vi "SkySparkCallForgetAcq.vi"(8 "error in (no error)":errorcluster, 11 "SkySparkDevice in":refnum<class "SkySparkDevice.lvclass">) -> (0 "error out":errorcluster, 2 "FGV_Cluster Output":T1, 3 "SkySparkDevice out":refnum<class "SkySparkDevice.lvclass">)   [LabVIEW 2020, in "SkySparkDevice.lvclass"]
uses:
  SkySparkDevice.lvclass
  FGV_TypeDef.ctl
  FGVFunctionTypeDef.ctl
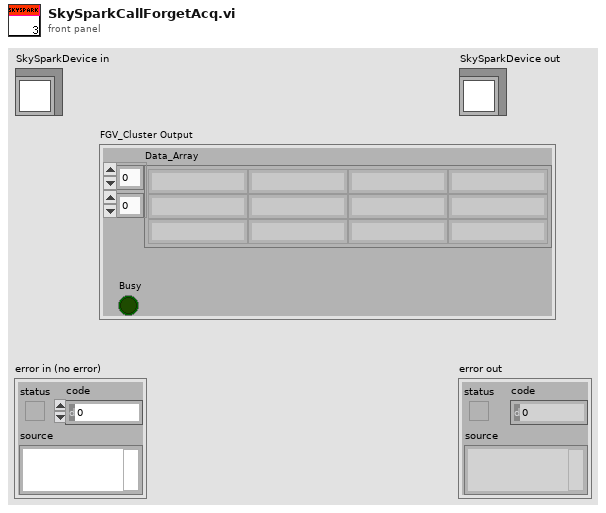
[diagram p1: front panel]
types:
  T1 = typedef "SkySparkDevice.lvclass/FGV_TypeDef.ctl" = cluster{"Data_Array":string[][], "Busy":bool}
  T2 = typedef "SkySparkDevice.lvclass/FGVFunctionTypeDef.ctl" = enum16{"Clear", "Write", "Read"}
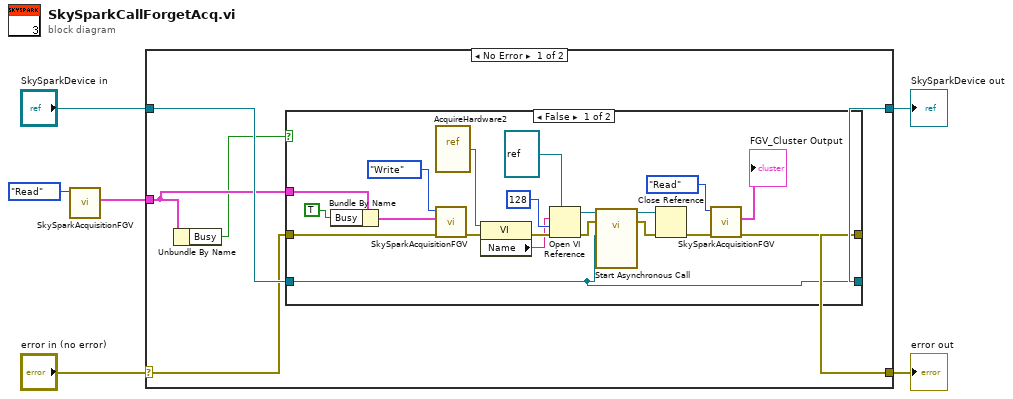
[diagram p0: block diagram]
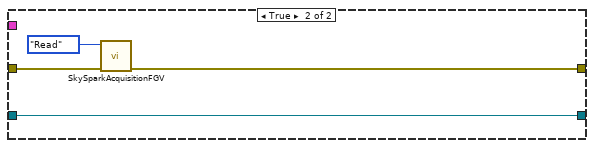
[diagram p2: hidden frame]
diagram:
  n1 = call "SkySparkAcquisitionFGV.vi"("Function"=FGVFunctionTypeDef."Read") -> ("FGV_Cluster Output"=w1:T1)  [unwired: 9 in, 1 out]
  n2 = case shown="No Error" "error in (no error)" {
    selector: "error in (no error)" -> [w10 w38]
    tunnel: [w9 w38] -> w5
    tunnel: [w11 w37] -> w3
    tunnel: "SkySparkDevice in" -> [w12 w37]
    tunnel: w1 -> [w8 _]
    frame No Error {
      n3 = Unbundle By Name(w8) -> ("Busy"=w7:bool)
      n4 = case shown="False" w7 {
        tunnel: w12 -> [w15 w33]
        tunnel: [w15 w33] -> w11
        tunnel: w10 -> [w24 w35]
        tunnel: [w21 w34] -> w9
        tunnel: w8 -> [w32 _]
        frame False {
          n5 = Bundle By Name(cluster=w32, "Busy"=TRUE) -> (w30:T1)
          n6 = vi-ref "AcquireHardware2.vi"() -> (w19:refnum<vi>)
          n7 = call "SkySparkAcquisitionFGV.vi"("error in (no error)"=w24, "FGV_Cluster Input"=w30, "Function"=FGVFunctionTypeDef."Write") -> ("error out"=w28:errorcluster)  [unwired: 7 in, 1 out]
          n8 = property class="VI"(reference=w19, error in=w28) -> (error out=w26:errorcluster, "Name"=w25:string)  [unwired: 1 out]
          n9 = Open VI Reference(type specifier VI Refnum (for type only)=refnum<vi> refnum, vi path=w25, options=128, error in (no error)=w26) -> (vi reference=w17:refnum<vi>, error out=w14:errorcluster)  [unwired: 2 in]
          n10 = call-by-ref "Start Asynchronous Call"(reference=w17, error in=w14, "SkySparkDevice in"=w15) -> (reference out=w18:refnum<vi>, error out=w13:errorcluster)  [unwired: 9 in, 2 out]
          n11 = Close Reference(reference=w18, error in (no error)=w13) -> (error out=w22:errorcluster)
          n12 = call "SkySparkAcquisitionFGV.vi"("error in (no error)"=w22, "Function"=FGVFunctionTypeDef."Read") -> ("error out"=w21:errorcluster, "FGV_Cluster Output"=→"FGV_Cluster Output":T1)  [unwired: 8 in]
        }
        frame True {
          n13 = call "SkySparkAcquisitionFGV.vi"("error in (no error)"=w35, "Function"=FGVFunctionTypeDef."Read") -> ("error out"=w34:errorcluster)  [unwired: 8 in, 1 out]
        }
      }
    }
    frame Error {
    }
  }
  "error out" <- w5
  "SkySparkDevice out" <- w3
